vi "Engine-Event-MouseButtonUp.vi"(4 "Position":T1, 6 "Button":u8, 7 "Clicks":u8, 8 "error in (no error)":errorcluster, 9 "Which":T2, 10 "Timestamp":u64, 11 "GLF Window in":refnum<class "Window.lvclass">) -> (0 "error out":errorcluster, 3 "GLF Window out":refnum<class "Window.lvclass">)   [LabVIEW 2020, in "GLF.lvlib" / "Window.lvclass"]
uses:
  Window.lvclass
  Window.lvclass/Window.ctl
  WindowEventInterface/WindowEventInterface.lvclass
  <vilib>/Saukko/LV SDL3/Sources/SDL3/Mouse/MouseID--integer.ctl
  <vilib>/Saukko/LV SDL3/Sources/SDL3/Mouse/Mouse.lvlib
  <vilib>/Saukko/LV SDL3/Sources/SDL3/Rect/FPoint--cluster.ctl
  <vilib>/Saukko/LV SDL3/Sources/SDL3/Rect/Rect.lvlib
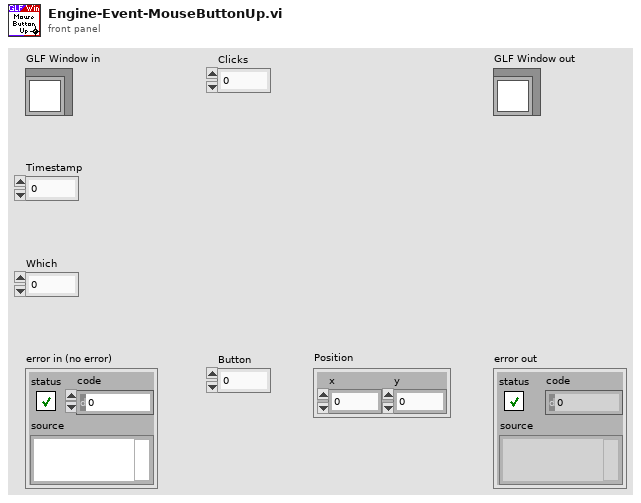
[diagram p1: front panel]
types:
  T1 = typedef "SDL3.lvlib/Rect.lvlib/FPoint--cluster.ctl" = cluster{"x":sgl, "y":sgl}
  T2 = typedef "SDL3.lvlib/Mouse.lvlib/MouseID--integer.ctl" = u32
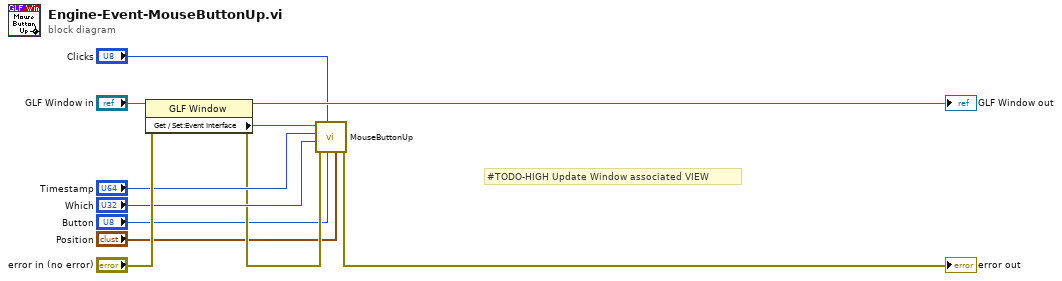
[diagram p0: block diagram]
diagram:
  # "#TODO-HIGH Update Window associated VIEW"
  n1 = property class="GLF Window"(reference="GLF Window in", error in="error in (no error)") -> (reference out=→"GLF Window out":refnum<class "Window.lvclass">, error out=w4:errorcluster, "Get / Set:Event Interface"=w8:refnum<class "WindowEventInterface.lvclass">)
  n2 = call-dynamic "MouseButtonUp.vi"("Position"="Position", "Button"="Button", "Clicks"="Clicks", "error in (no error)"=w4, "Which"="Which", "Timestamp"="Timestamp", "WindowEventInterface in"=w8) -> ("error out"=→"error out":errorcluster)  [unwired: 4 in]
